vi "Configuration File Handler.vi"(8 "error in":errorcluster, 10 "selected configuration file":path, 11 "configuration file page data":T1 {"custom device ref" format="%.0x"}) -> (0 "error out":errorcluster, 3 "configuration file page data out":T1 {"custom device ref" format="%.0x"})   [LabVIEW 2020, in "AIM ARINC 664 System Explorer.lvlib" / "Implementation.lvlib"]
uses:
  Implementation.lvlib
  Types/Browse Button.ctl
  Types/Path Control.ctl
  Import/AIM ARINC 664 Import.lvlib
  Scripting/AIM ARINC 664 Scripting.lvlib
  <vilib>/NI VeriStand/Custom Device API/Custom Device Item Ref.ctl
  <vilib>/NI VeriStand/Custom Device API/Custom Device API.lvlib
  Types/Configuration File Page Data.ctl
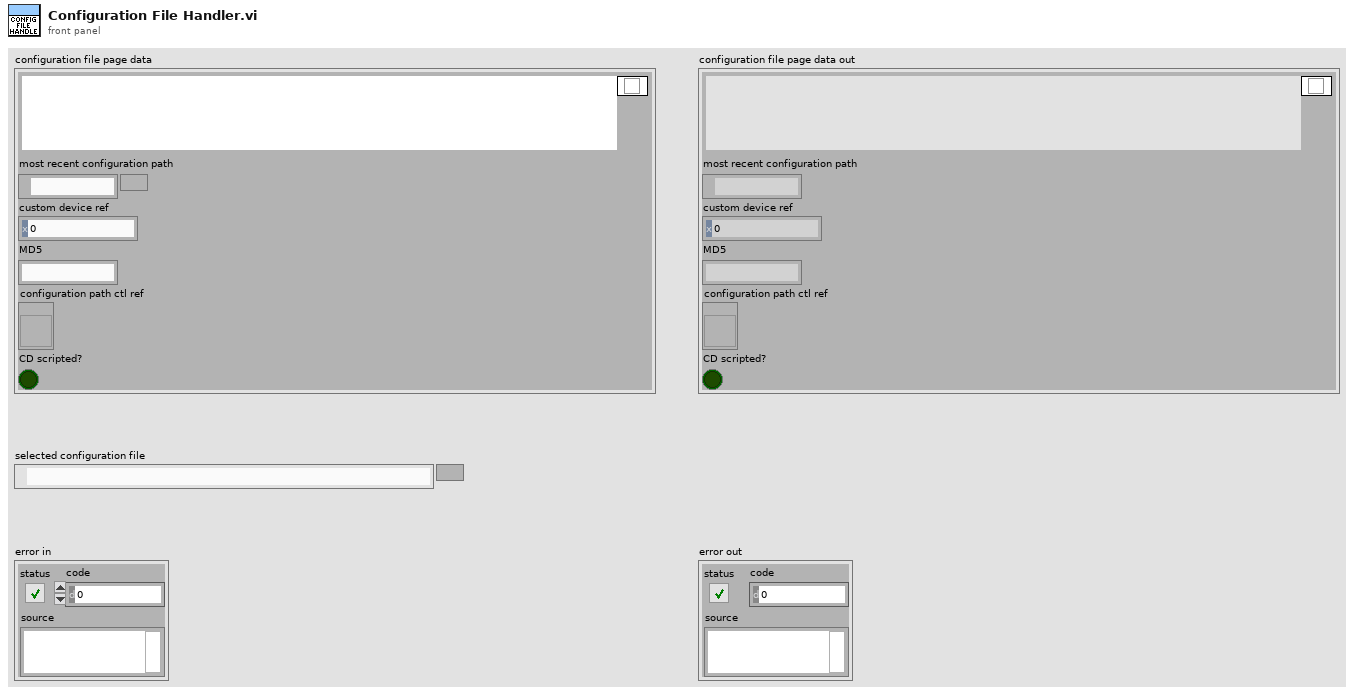
[diagram p1: front panel]
types:
  T1 = typedef "AIM ARINC 664 System Explorer.lvlib/Implementation.lvlib/Configuration File Page Data.ctl" = cluster{"Parameters":T2, "most recent configuration path":path, "custom device ref":T4, "MD5":string, "configuration path ctl ref":refnum<vi>, "CD scripted?":bool}
  T2 = typedef "AIM ARINC 664 System Explorer.lvlib/Implementation.lvlib/Path Control.ctl" = cluster{"file path":path, "Browse":T3}
  T3 = typedef "AIM ARINC 664 System Explorer.lvlib/Implementation.lvlib/Browse Button.ctl" = bool
  T4 = typedef "Custom Device API.lvlib/Custom Device Item Ref.ctl" = u64
  T5 = typedef "AIM ARINC 664 Import.lvlib/Board Top Level Configuration.ctl" = cluster{"boardSetup":T6, "portConfiguration":T7[]}
  T6 = typedef "AIM ARINC 664 Import.lvlib/board_setup.ctl" = cluster{"boardId":u32, "portSpeed":u32, "portConfig":u32}
  T7 = typedef "AIM ARINC 664 Import.lvlib/port_configuration.ctl" = cluster{"portSetup":T8, "Tx_Generic":T9[], "Rx_Monitor":cluster{"DefaultCronoMode":u32, "GlbMonBufferSizeIn":u32, "CaptureMode":u32, "MaxFileSizeMB":u32, "Strobe":u32, "TriggerPosition":u32}[], "Tx_UDP":cluster{"tx_udp_setup":T14, "commPorts":T15[], "sapPorts":T19[]}[], "Rx_UDP":cluster{"Tx_UDP":T20, "commPorts":T21[], "sapPorts":T22[]}[]}
  T8 = typedef "AIM ARINC 664 Import.lvlib/port_setup.ctl" = cluster{"portId":u32, "portMap":u32}
  T9 = typedef "AIM ARINC 664 Import.lvlib/session_tx_generic.ctl" = cluster{"tx_generic_setup":T10, "Frame Headers":T11[]}
  T10 = typedef "AIM ARINC 664 Import.lvlib/tx_generic_setup.ctl" = cluster{"QueueSizeIn":u32, "Count":i32, "StartMode":i32}
  T11 = typedef "AIM ARINC 664 Import.lvlib/frame_tx_generic.ctl" = cluster{"ID":string, "Frame header":cluster{"FrameStartMode":i32, "InterFrameGap":i32, "PacketGroupWaitTime":i32, "NetSelect":i32, "PayloadBufferMode":i32, "PayloadGenerationMode":i32, "PhysErrorInjection":i32, "PreambleCount":i32, "SequenceNumberInit":T12, "SequenceNumberOffset":T13, "Skew":i32}}
  T12 = typedef "AIM ARINC 664 Import.lvlib/frame_tx_generic_seqNumberInit.ctl" = i32
  T13 = typedef "AIM ARINC 664 Import.lvlib/frame_tx_generic_seqNumberOffset.ctl" = i32
  T14 = typedef "AIM ARINC 664 Import.lvlib/tx_udp_setup.ctl" = cluster{"VlId":i32, "Bag":i32, "NetSelect":i32, "domainID":u8, "sideID":u8, "locationID":u8, "interfaceID":u8, "NumOfSubVl":u16, "Skew":u32, "MaxFrameLength":u32, "FrameBufferSize":u32}
  T15 = typedef "AIM ARINC 664 Import.lvlib/port_tx_udp_comm.ctl" = cluster{"ID":string, "partitionID":u8, "UdpSrcPort":u16, "UdpDstPort":u16, "PortType":enum16{"FDX_UDP_SAMPLING", "FDX_UDP_QUEUING"}, "SubVIId":u32, "UdpNumBufMessages":u32, "UdpMaxMessageSize":u32, "UdpSamplingRate":u32, "Parameters":T16[]}
  T16 = typedef "AIM ARINC 664 Import.lvlib/frame_parameter.ctl" = cluster{"name":string, "default value":dbl, "unit":string, "Parameter":T17}
  T17 = typedef "AIM ARINC 664 Import.lvlib/frame_parameter_definition.ctl" = cluster{"start index":i32, "size":i32, "encoding":T18, "signed":bool, "scale multiplier":dbl, "scale offset":dbl}
  T18 = typedef "Encoding and Decoding.lvlib/Encoding.ctl" = enum16{"BNR", "BCD", "Discrete"}
  T19 = typedef "AIM ARINC 664 Import.lvlib/port_tx_udp_sap.ctl" = cluster{"ID":string, "SubVlId":u8, "UdpSrcPort":u16, "UdpNumBufMessages":u32, "UdpMaxMessageSize":u32, "partitionID":u8, "domainID":u8, "sideID":u8, "locationID":u8, "interfaceID":u8, "Parameters":T16[]}
  T20 = typedef "AIM ARINC 664 Import.lvlib/rx_udp_setup.ctl" = cluster{"VerificationMode":u32, "Bag":u32, "Jitter":u32, "MaxFrameLength":u32, "MaxSkew":u32, "VLBufSize":u32, "FilterMode":u32, "FilterPosition":u32, "Padding":u32, "FilterMask":u32, "FilterData":u32, "MinFrameLength":u32, "VlId":u16, "VLRange":u32}
  T21 = typedef "AIM ARINC 664 Import.lvlib/port_rx_udp_comm.ctl" = cluster{"ID":string, "domainID":u8, "sideID":u8, "locationID":u8, "partitionID":u8, "UdpSrcPort":u16, "UdpDstPort":u16, "PortType":enum16{"FDX_UDP_SAMPLING", "FDX_UDP_QUEUING"}, "SubVIId":u32, "UdpNumBufMessages":u32, "UdpMaxMessageSize":u32, "UdpSamplingRate":u32, "Parameters":T16[]}
  T22 = typedef "AIM ARINC 664 Import.lvlib/port_rx_udp_sap.ctl" = cluster{"ID":string, "UdpDstPort":u16, "UdpNumBufMessages":u32, "UdpMaxMessageSize":u32, "Parameters":T16[]}
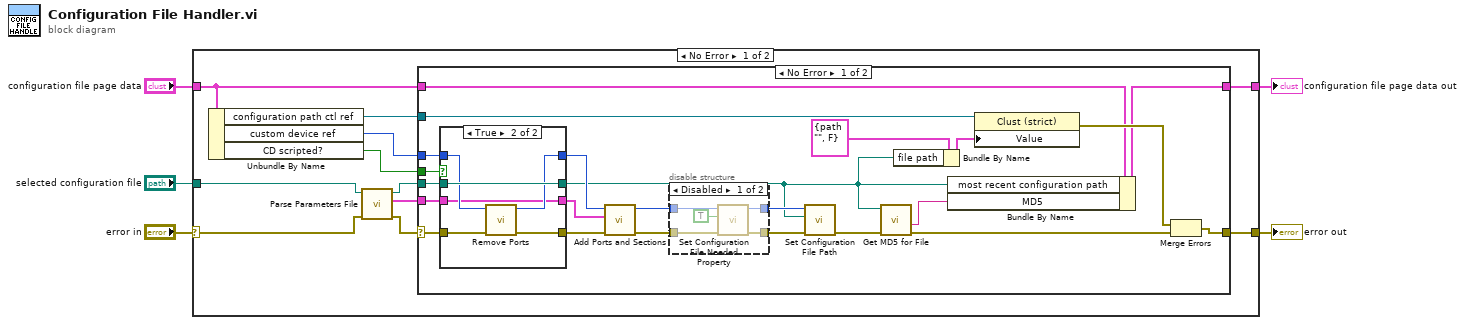
[diagram p0: block diagram]
diagram:
  n1 = case shown="No Error" "error in" {
    selector: "error in" -> [w9 w59]
    tunnel: "configuration file page data" -> [w16 w60]
    tunnel: "selected configuration file" -> [w10 _]
    tunnel: [w12 w60] -> w2
    tunnel: [w15 w59] -> w1
    frame No Error {
      n2 = Unbundle By Name(w16) -> ("configuration path ctl ref"=w14:refnum<vi>, "custom device ref"=w13:T4, "CD scripted?"=w11:bool)
      n3 = call "Parse Parameters File.vi"("error in"=w9, "path to XML document"=w10) -> ("error out"=w6:errorcluster, "board configuration out"=w7:T5, "path to XML document out"=w8:path)  [unwired: 7 in]
      n4 = case shown="No Error" w6 {
        selector: w6 -> [w17 w58]
        tunnel: w16 -> [w38 w57]
        tunnel: [w37 w58] -> w15
        tunnel: w14 -> [w36 _]
        tunnel: w13 -> [w32 _]
        tunnel: [w30 w57] -> w12
        tunnel: w11 -> [w29 _]
        tunnel: w8 -> [w22 _]
        tunnel: w7 -> [w18 _]
        frame No Error {
          n5 = case shown="True" w29 {
            tunnel: w22 -> [w49 w56]
            tunnel: w17 -> [w50 w55]
            tunnel: [w50 w54] -> w20
            tunnel: [w49 w56] -> w21
            tunnel: w32 -> [w48 w53]
            tunnel: [w48 w52] -> w31
            tunnel: [w47 w51] -> w19
            tunnel: w18 -> [w47 w51]
            frame False {
            }
            frame True {
              n6 = call "Remove Ports.vi"("error in"=w55, "Custom device Ref"=w53) -> ("error out"=w54:errorcluster, "Custom device Ref out"=w52:T4)  [unwired: 8 in]
            }
          }
          n7 = call "Add Ports and Sections.vi"("error in"=w20, "board configuration in"=w19, "custom device ref"=w31) -> ("error out"=w23:errorcluster, "custom device ref out"=w24:T4)  [unwired: 7 in]
          n8 = disable-structure shown="Disabled" {
            disable-tunnel: [w43 w46] -> w28
            disable-tunnel: [w42 w45] -> w25
            disable-tunnel: w24 -> [w41 w45]
            disable-tunnel: w23 -> [w40 w46]
            frame Disabled {
              n9 = call "Set Configuration File Needed Property.vi"("error in"=w40, "needed?"=TRUE, "custom device ref in"=w41) -> ("error out"=w43:errorcluster, "custom device ref out"=w42:T4)  [unwired: 7 in]
            }
            frame Enabled {
            }
          }
          n10 = call "Set Configuration File Path.vi"("error in"=w28, "configuration file path"=w21, "custom device ref in"=w25) -> ("error out"=w26:errorcluster)  [unwired: 7 in, 1 out]
          n11 = call "Get MD5 for File.vi"("error in"=w26, "Path"=w21) -> ("error out"=w27:errorcluster, "MD5"=w35:string)  [unwired: 8 in]
          n12 = Bundle By Name(cluster=T2 {"file path"=path "", "Browse"=FALSE} ("Path"), "file path"=w21) -> (w33:T2)
          n13 = Bundle By Name(cluster=w38, "most recent configuration path"=w21, "MD5"=w35) -> (w30:T1)
          n14 = property class="Clust (strict)"(reference=w36, "Value"=w33) -> (error out=w39:errorcluster)  [unwired: 1 in, 1 out]
          n15 = Merge Errors(w39, w27) -> (w37:errorcluster)
        }
        frame Error {
          # "If error happens, keep the previous configuration. It can be empty\nor previous configuration"
        }
      }
    }
    frame Error {
    }
  }
  "configuration file page data out" <- w2
  "error out" <- w1
